vi "Control_Valves_and_Pumps.vi"(8 "Set state:":bool, 10 "Device":T1, 11 "Mode of Operation":bool) -> ()   [LabVIEW 2011]
uses:
  SubVI/Valve_Pump.ctl
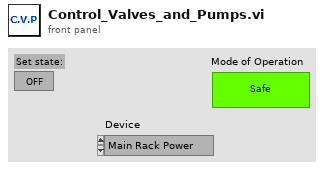
[diagram p1: front panel]
types:
  T1 = typedef "Valve_Pump.ctl" = enum16{"Main Rack Power", "Pump Power", "Valve Power", "V4", "V5", "V6", "V7", "V8", "V9", "V10", "V11", "V12", "V13", "V14", "V15", "V18", "V19", "V20", "V21", "V22", "V23", "V24", "V25", "V26", "V27", "V28", "V29", "V30", "V31", "V32", "V33", "V34", "Pump A", "Pump B", "Pump C", "Pump D"}
  T2 = typedef "Address.ctl" = cluster{"Main":i32, "Ch.":i32, "Sub":i32, "Port Name":string}
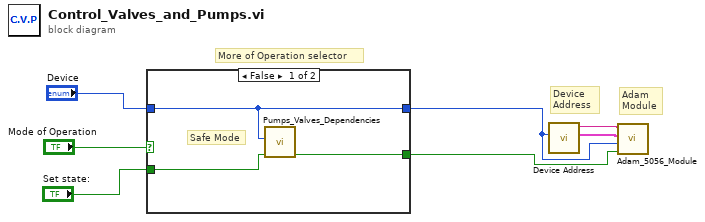
[diagram p0: block diagram]
diagram:
  # "Adam \nModule"
  # "Device\nAddress"
  # "More of Operation selector"
  n1 = case shown="False" "Mode of Operation" {
    tunnel: "Device" -> [w8 w12]
    tunnel: "Set state:" -> [w10 w11]
    tunnel: [w9 w11] -> w4
    tunnel: [w8 w12] -> w1
    frame False {
      # "Safe Mode"
      n2 = call "Pumps_Valves_Dependencies.vi"("Set state:"=w10, "Device"=w8) -> ("State"=w9:bool)  [unwired: 9 in]
    }
    frame True {
      # "Maintenance Mode"
    }
  }
  n3 = call "Device Address.vi"("Device"=w1) -> ("Address (all reqd.)"=w3:T2, "Channel Name"=w2:string)  [unwired: 9 in]
  n4 = call "Adam_5056_Module.vi"("Set state:"=w4, "Device"=w1, "Address (all reqd.)"=w3, "Channel Name"=w2) -> ()  [unwired: 8 in]
